vi "BB_CameraInit.vi"(11 "Camera IP In":string) -> (3 "Camera IP Out":string)   [LabVIEW 2015]
uses:
  <vilib>/Rock Robotics/WPI/Camera/WPI_CameraWhite Balance Values.ctl
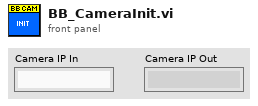
[diagram p1: front panel]
types:
  T1 = typedef "WPI_CameraWhite Balance Values.ctl" = enum16{"Auto", "Fixed indoor", "Fixed outdoor 1", "Fixed outdoor 2", "Fixed fluorescent 1", "Fixed fluorescent 2", "Hold current", "Custom"}
  T2 = typedef "WPI_CameraDevRef.ctl" = cluster{"Camera Address":string, "CameraStatus":errorcluster}
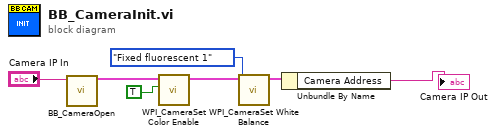
[diagram p0: block diagram]
diagram:
  n1 = call "BB_CameraOpen.vi"("Camera Address"="Camera IP In") -> ("CameraDevRef"=w1:T2)  [unwired: 9 in, 1 out]
  n2 = call <vilib>:"WPI_CameraSet Color Enable.vi"("Color Enabled"=TRUE, "CameraDevRef"=w1) -> ("CameraDevRef Out"=w3:T2)  [unwired: 8 in, 1 out]
  n3 = call <vilib>:"WPI_CameraSet White Balance.vi"("White Balance"=WPI_CameraWhite_Balance_Values."Fixed fluorescent 1", "CameraDevRef"=w3) -> ("CameraDevRef Out"=w6:T2)  [unwired: 8 in, 1 out]
  n4 = Unbundle By Name(w6) -> ("Camera Address"=→"Camera IP Out":string)
